vi "ExcelOpen.vi"(8 "error in (no error)":errorcluster, 10 "File Path":path, 11 "ExcelFile in":refnum<class "PortableExcelFileManipulationOXML.lvclass">) -> (0 "error out":errorcluster, 3 "ExcelFile out":refnum<class "PortableExcelFileManipulationOXML.lvclass">)   [LabVIEW 2019, in "PortableExcelFileManipulationOXML.lvclass"]
doc: "Opens a Excel document from file. This allows for reading and writing functions to minipulate the object loaded into memory."
uses:
  PortableExcelFileManipulationOXML.lvclass
  H:/LV projects/ExpressionEvaluator/Excel/ExcelManipulation.dll
  ExcelManipulation.dll
  PortableExcelFileManipulationOXML.lvclass/PortableExcelFileManipulationOXML.ctl
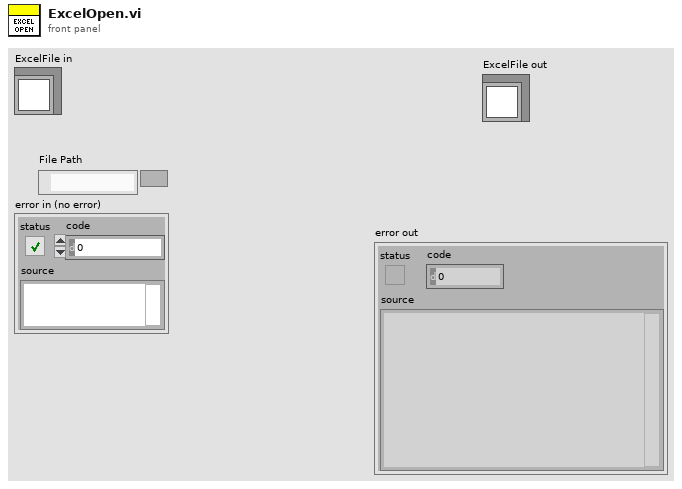
[diagram p1: front panel]
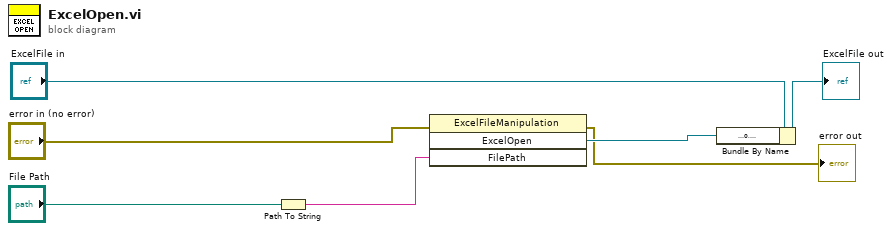
[diagram p0: block diagram]
diagram:
  n1 = Path To String(path="File Path") -> (string=w1:string)
  n2 = invoke class="ExcelFileManipulation" method="ExcelOpen"(error in="error in (no error)", "FilePath"=w1) -> (error out=→"error out":errorcluster, "ExcelOpen"=w5:refnum<k24>)  [unwired: 2 in, 2 out]
  n3 = Bundle By Name(cluster="ExcelFile in", "ExcelOpen"=w5) -> (→"ExcelFile out":refnum<class "PortableExcelFileManipulationOXML.lvclass">)
